vi "Send Refresh Rooms Status.vi"(6 "Room Service Map":T5(c390), 7 "Message Priority (Normal)":T6=enum."Normal", 8 "error in (no error)":errorcluster, 9 "Rooms List":T1[](array[typedef]), 10 "Room Size Details":T4[](array[typedef]), 11 "Message Enqueuer":refnum<class "Message Enqueuer.lvclass">) -> (0 "error out":errorcluster, 3 "Message Enqueuer out":refnum<class "Message Enqueuer.lvclass">)   [LabVIEW 2023, in "Rooms Manager Model.lvlib" / "Refresh Rooms Status Msg.lvclass"]
doc: "This VI sends the message to an actor."
uses:
  Refresh Rooms Status Msg.lvclass
  <vilib>/ActorFramework/Message Enqueuer/Message Enqueuer.lvclass
  <vilib>/ActorFramework/Message Enqueuer/Message Priority.ctl
  Room Service Types/Room Service Base/Room Service Base.lvclass
  Central Data Manager/Central Data Manager/Room Size Details.ctl
  Central Data Manager/Central Data Manager/Room Details.ctl
  Central Data Manager/Central Data Manager/Room Occupancy Status.ctl
  Central Data Manager/Central Data Manager/Guest Details.ctl
  C:/Program Files/National Instruments/LabVIEW 2023/vi.lib/ActorFramework/Message/Message.lvclass
  Refresh Rooms Status Msg.lvclass/Refresh Rooms Status Msg.ctl
  <vilib>/ActorFramework/Message Enqueuer/Message Enqueuer.lvclass/Message Enqueuer.ctl
  <vilib>/ActorFramework/Message Priority Queue/Priority Enqueue.vi
  Central Data Manager/Central Data Manager/Central Data Manager.lvclass
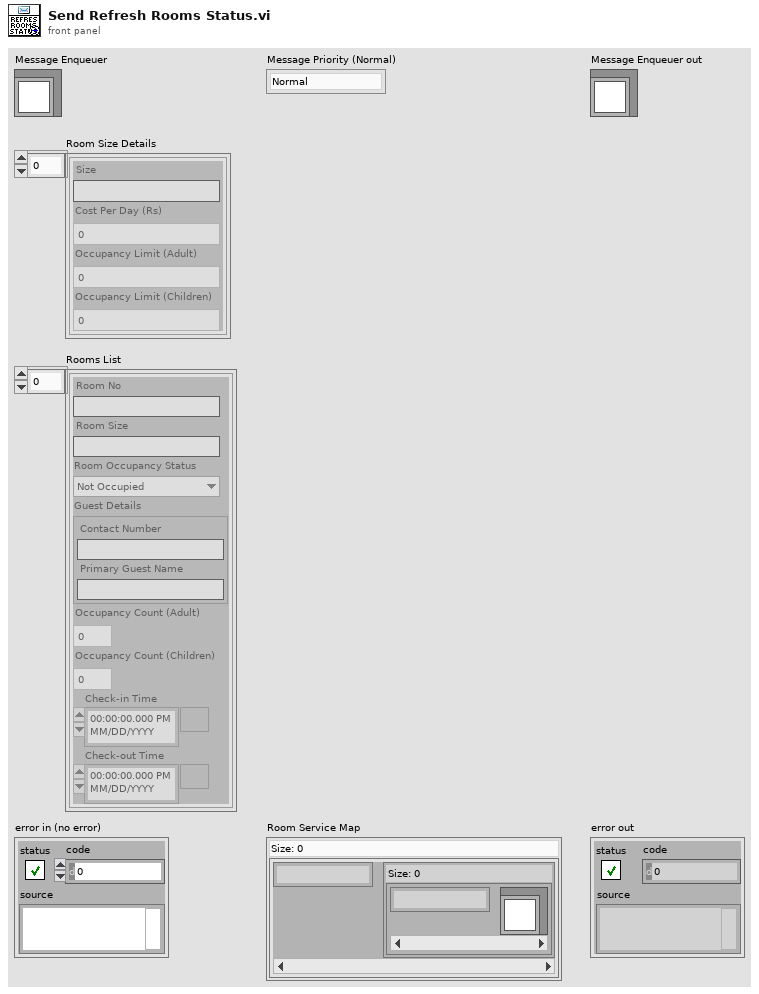
[diagram p1: front panel]
types:
  T1 = typedef "Central Data Manager.lvlib/Central Data Manager.lvclass/Room Details.ctl" = cluster{"Room No":string, "Room Size":string, "Room Occupancy Status":T2, "Guest Details":T3, "Occupancy Count (Adult)":u32, "Occupancy Count (Children)":u32, "Check-in Time":timestamp, "Check-out Time":timestamp}
  T2 = typedef "Central Data Manager.lvlib/Central Data Manager.lvclass/Room Occupancy Status.ctl" = enum16{"Not Occupied", "Occupied", "Under Maintainance", "Not Servicable"}
  T3 = typedef "Central Data Manager.lvlib/Central Data Manager.lvclass/Guest Details.ctl" = cluster{"Contact Number":string, "Primary Guest Name":string}
  T4 = typedef "Central Data Manager.lvlib/Central Data Manager.lvclass/Room Size Details.ctl" = cluster{"Size":string, "Cost Per Day (Rs)":u32, "Occupancy Limit (Adult)":u32, "Occupancy Limit (Children)":u32}
  T5 = map{string, map{string, refnum<class "Room Service Base.lvclass">}}
  T6 = typedef "Actor Framework.lvlib/Message Enqueuer.lvclass/Message Priority.ctl" = enum16{"Low", "Normal", "High"}
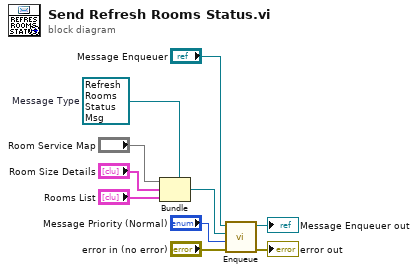
[diagram p0: block diagram]
diagram:
  w4 = refnum<class "Refresh Rooms Status Msg.lvclass"> refnum  # Message Type
  n1 = Bundle(cluster=w4, "Room Service Map", "Room Size Details", "Rooms List") -> (w5:refnum<class "Refresh Rooms Status Msg.lvclass">)
  n2 = call <vilib>:"Enqueue.vi"("error in (no error)"="error in (no error)", "Message Priority (Normal)"="Message Priority (Normal)", "Message"=w5, "Message Enqueuer in"="Message Enqueuer") -> ("error out"=→"error out":errorcluster, "Message Enqueuer out"=→"Message Enqueuer out":refnum<class "Message Enqueuer.lvclass">)  [unwired: 6 in]
